vi "3.5.vi"(1 "数值":dbl) -> (0 "数值 2":dbl)   [LabVIEW 2017]
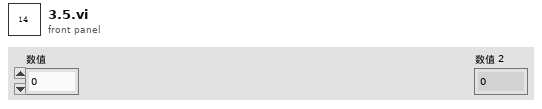
[diagram p1: front panel]
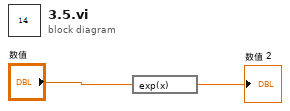
[diagram p0: block diagram]
diagram:
  n1 = expression code="exp(x)"("数值") -> (→"数值 2":dbl)
